vi "RadioSelection.vi"(10 "error in (no error)":errorcluster, 11 "Group":u8) -> (2 "error out":errorcluster, 3 "RadioSelection out":refnum<class "MGI_RadioSelection.lvclass">)   [LabVIEW 2016, in "MGI_RadioSelection.lvclass"]
doc: "Radio selection mimics the action of a radio button. Only one item in the Radio Group can be selected at a time. The Radio group is defined by the Group input. When a item in a radio group is selected, first a MenuItem Clicked event is generated with an \"Unchecked\" message indicating what item has been unchecked. Next a MenuItem Clicked event is generated with a \"Clicked\" message indicating the new item that has been checked. The Unchecked message will always come before the Clicked message. If a checked item is clicked again by the user, the click is ignored.\n\nNote: Groups only apply to a common level of menus. For example, Item 1 and Item 2 are in Radio Group 1. Item 3 has a submenu containing TextA and TextB. TextA and TextB have a radio Group 1. When Item 1 or Item 2 are clicked, it does not affect TextA or TextB, since they are not on the same menu level.\n\nAuthored by Derek E. Trepanier\nsupport@mooregoodideas.com\nwww.mooregoodideas.com\n\nCopyright (c) 2012, Moore Good Ideas, Inc.\n\nAll rights reserved.\n\nRedistribution and use in source and binary forms, with or without modification, are permitted provided that the following conditions are met:\n\n * Redistributions of source code must retain the above copyright notice, this list of conditions and the following disclaimer.\n * Redistributions in binary form must reproduce the above copyright notice, this list of conditions and the following disclaimer in the documentation and/or other materials provided with the distribution.\n * Neither the name of Moore Good Ideas, Inc. nor the names of its contributors may be used to endorse or promote products derived from this software without specific prior written permission.\n\nTHIS SOFTWARE IS PROVIDED BY THE COPYRIGHT HOLDERS AND CONTRIBUTORS \"AS IS\" AND ANY EXPRESS OR IMPLIED WARRANTIES, INCLUDING, BUT NOT LIMITED TO, THE IMPLIED WARRANTIES OF MERCHANTABILITY AND FITNESS FOR A PARTICULAR PURPOSE ARE DISCLAIMED. IN NO EVENT SHALL THE COPYRIGHT OWNER OR CONTRIBUTORS BE LIABLE FOR ANY DIRECT, INDIRECT, INCIDENTAL, SPECIAL, EXEMPLARY, OR CONSEQUENTIAL DAMAGES (INCLUDING, BUT NOT LIMITED TO, PROCUREMENT OF SUBSTITUTE GOODS OR SERVICES; LOSS OF USE, DATA, OR PROFITS; OR BUSINESS INTERRUPTION) HOWEVER CAUSED AND ON ANY THEORY OF LIABILITY, WHETHER IN CONTRACT, STRICT LIABILITY, OR TORT (INCLUDING NEGLIGENCE OR OTHERWISE) ARISING IN ANY WAY OUT OF THE USE OF THIS SOFTWARE, EVEN IF ADVISED OF THE POSSIBILITY OF SUCH DAMAGE."
uses:
  <userlib>/_MGI/Menu Building/SelectionType/RadioSelection/MGI_RadioSelection.lvclass
  <userlib>/_MGI/Menu Building/SelectionType/RadioSelection/MGI_RadioSelection.lvclass/MGI_RadioSelection.ctl
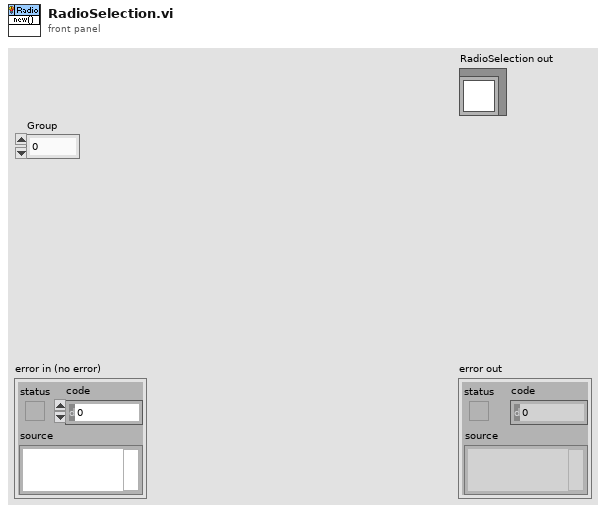
[diagram p1: front panel]
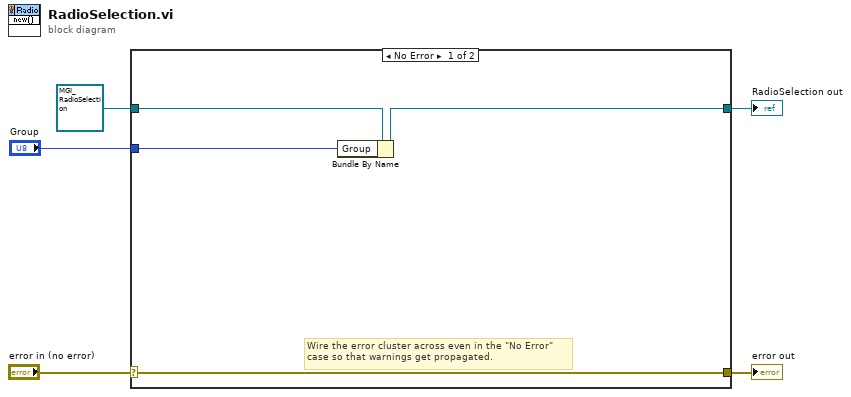
[diagram p0: block diagram]
diagram:
  n1 = case shown="No Error" "error in (no error)" {
    selector: "error in (no error)" -> [w8 w11]
    tunnel: [w8 w11] -> w4
    tunnel: [w7 w10] -> w2
    tunnel: refnum<class "MGI_RadioSelection.lvclass"> refnum ("RadioSelection in") -> [w9 w10]
    tunnel: "Group" -> [w6 _]
    frame No Error {
      # "Wire the error cluster across even in the \"No Error\"\ncase so that warnings get propagated."
      n2 = Bundle By Name(cluster=w9, "Group"=w6) -> (w7:refnum<class "MGI_RadioSelection.lvclass">)
    }
    frame Error {
    }
  }
  "error out" <- w4
  "RadioSelection out" <- w2
